vi "MPC_Sim_2.vi"() -> ()   [LabVIEW 2018]
uses:
  <vilib>/Simulation/Scripting/Companion Diagram/SimConfigNode/SimParams.ctl
  <vilib>/Simulation/Scripting/Companion Diagram/SimConfigNode/_simSolvers.ctl
  <vilib>/Simulation/Implementation/Shared/SIMSCR Execution Mode.ctl
  <vilib>/Simulation/Param Hierarchy/Typedefs/SIMPH Param Control Actions.ctl
  <vilib>/Simulation/Scripting/Editor Utilities/SIM subVI tag data.ctl
  <vilib>/Simulation/Scripting/Editor Utilities/SIM subVI execution type.ctl
  <vilib>/Simulation/Implementation/Shared/NILVSim_ParamChanged.vi
  <vilib>/Simulation/Implementation/Shared/NILVSIM_BeginStep.vi
  <vilib>/Simulation/Utility/Implementation/SIM Halt.vi
  <vilib>/Simulation/SignalArithmetic/Implementation/NILVSim Gain.llb/SIM Gain (vector).vi
  <vilib>/Simulation/Utility/Implementation/NILVSim Memory.llb/NILVSim Memory (core).vi
  <vilib>/Simulation/DiscreteLinear/Implementation/NILVSim Discrete State Space Buffered.llb/SIM Discrete State Space Distributor (SISO CD).vi
  <vilib>/Simulation/SignalArithmetic/Implementation/NILVSim Gain.llb/SIM Gain (scalar).vi
  <vilib>/Simulation/SignalDisplay/Implementation/NILVSim Time Waveform.llb/SIM Time Waveform (scalar).vi
  <vilib>/Simulation/Implementation/Shared/SIM Fire Discrete SubVI.vi
  <vilib>/Simulation/SignalDisplay/Implementation/NILVSim Time Waveform.llb/SIM Time Waveform (vector).vi
  <vilib>/Simulation/DiscreteLinear/Implementation/NILVSim Discrete State Space Buffered.llb/SIM Discrete State Space Collector (SISO CD).vi
  <vilib>/Simulation/Implementation/Shared/NILVSim_Manager.vi
  <vilib>/Utility/error.llb/Clear Errors.vi
  <vilib>/Simulation/Implementation/Shared/NILVSim_FinalizeModel.vi
  <vilib>/Simulation/Implementation/Shared/SIM Fire Discrete SubVI (Core).vi
  <vilib>/imath/engines/lvmath2/RunTimeEngine/IndexRead/NIMS M(S,S).vi
  <instcachedir>/0/NIMS M(S,S)_AC51E74150A542F7991B9634C66F3096.lvgen/NIMS M(S,S)_AC51E74150A542F7991B9634C66F3096_000.vi
  <vilib>/imath/engines/lvmath2/RunTimeEngine/IndexRead/NIMS V(S).vi
  <instcachedir>/0/NIMS V(S)_0488751826AF41519A22953C041130DC.lvgen/NIMS V(S)_0488751826AF41519A22953C041130DC_000.vi
  <vilib>/imath/engines/lvmath2/RunTimeEngine/IndexReplace/NIMS M(S,S)=S.vi
  <instcachedir>/0/NIMS M(S,S)=S_5DAF17B45D8A4C8588C7CF468644990A.lvgen/NIMS M(S,S)=S_5DAF17B45D8A4C8588C7CF468644990A_000.vi
  <vilib>/imath/engines/lvmath2/RunTimeEngine/ErrorHandling/NIMS_Create Error From Enums.vi
  <vilib>/imath/engines/lvmath/Plug In/Control Design/BuiltInFunctions/ss/NIMS_CD_ss(A,B,C,D).vi
  <vilib>/imath/engines/lvmath2/RunTimeEngine/NodeEndStatement/NIMS_NodeEndStatement_Output.vi
  <instcachedir>/0/NIMS_NodeEndStatement_Output_53EC0D466D134D7ABD903AC30B43404B.lvgen/NIMS_NodeEndStatement_Output_53EC0D466D134D7ABD903AC30B43404B_001.vi
  <instcachedir>/0/NIMS_NodeEndStatement_Output_53EC0D466D134D7ABD903AC30B43404B.lvgen/NIMS_NodeEndStatement_Output_53EC0D466D134D7ABD903AC30B43404B_011.vi
  <vilib>/imath/engines/lvmath2/RunTimeEngine/ErrorHandling/NIMS_Finalize Error.vi
  <vilib>/addons/Control Design/_Model Conversions/Continuous and Discrete.llb/Continuous and Discrete SubVI/cd_Convert Continuous to Discrete (SS).vi
  <vilib>/addons/Control Design/_MPC/Build Controller/CD Create MPC Controller (Barrier).vi
  <vilib>/imath/engines/lvmath2/RunTimeEngine/Managers/WorkSpace/UID Generator.vi
  <vilib>/imath/engines/lvmath2/RunTimeEngine/RangeToken/NIMS_Range.vi
  <instcachedir>/0/NIMS_Range_846134F467D14A349F7C6CCEF459CDB2.lvgen/NIMS_Range_846134F467D14A349F7C6CCEF459CDB2_000.vi
  <vilib>/imath/engines/lvmath2/RunTimeEngine/RunTimeType/NIMS_RunTimeType_From StrictType (excl LVString).vi
  <instcachedir>/0/NIMS_RunTimeType_From StrictType (excl LVString)_E7E34A65C99947108168652BAD14964D.lvgen/NIMS_RunTimeType_From StrictType (excl LVString)_E7E34A65C99947108168652BAD14964D_000.vi
  <vilib>/imathl/engines/lvmath/Functions/Error Handling/Create Error.vi
  <vilib>/imath/engines/lvmath2/RunTimeEngine/LocalVariableDefStatement/MC_LocalVariableDefStatement_Display.vi
  <vilib>/imath/engines/lvmath2/RunTimeEngine/BuiltInFunctions/square/NIMS_square.vi
  <instcachedir>/0/NIMS_square_8BE126634BDB49EE87F69273AACFE816.lvgen/NIMS_square_8BE126634BDB49EE87F69273AACFE816_001.vi
  <vilib>/imath/engines/lvmath2/RunTimeEngine/Managers/SymbolTable/Clear UID.vi
  <instcachedir>/0/NIMS_NodeEndStatement_Output_53EC0D466D134D7ABD903AC30B43404B.lvgen/NIMS_NodeEndStatement_Output_53EC0D466D134D7ABD903AC30B43404B_005.vi
  <vilib>/Simulation/Implementation/Shared/SIM Unbundle Sim Info.vi
  <vilib>/Simulation/Implementation/Shared/NILVSim_Initialize.vi
  <vilib>/Simulation/Utility/Implementation/NILVSim Get Time and IsAcceptedStep.vi
  <vilib>/addons/Control Design/_MPC/Reference Profile/CD Step Forward MPC Window.vi
  <vilib>/addons/Control Design/_MPC/Implement Controller/CD Implement MPC Controller.vi
  <vilib>/addons/Control Design/_MPC/Implement Controller/CD Implement MPC Controller (MIMO).vi
  <vilib>/Simulation/Implementation/Shared/SIMSH Read Queue.vi
  <vilib>/Simulation/Implementation/Shared/NILVSim_GetModelError.vi
  <vilib>/Simulation/Implementation/Shared/SIM Bundle Sim Info.vi
  <vilib>/Simulation/Scripting/Companion Diagram/SimConfigNode/SimDog.xnode
  <vilib>/addons/Control Design/_Model Construction/Model Typedefs.llb/CD State Space Model (MIMO).ctl
  <vilib>/addons/Control Design/_Model Construction/Model Typedefs.llb/CD General Elements.ctl
  <vilib>/Simulation/Implementation/XNodeFramework/SimXNode/SimX.xnode
  <vilib>/addons/Control Design/_Model Construction/NI_LinSys_Model Typedefs.lvlib
  <vilib>/addons/Control Design/_MPC/NI_CD_MPC.lvlib
  <vilib>/addons/Control Design/_Model Conversions/NI_CD_Continuous and Discrete.lvlib
  <vilib>/Simulation/DiscreteLinear/Implementation/NILVSim Discrete State Space Buffered.llb/SIM Discrete State Space Buffered (SISO CD).vi
  <vilib>/Simulation/Implementation/Shared/NI_SIM_Implementation.lvlib
  <vilib>/imath/engines/lvmath2/RunTimeEngine/Managers/SymbolTable/NIMS_WorkSpace.lvlib
panel:
  in  "Sampling Time":dbl=0.05 format="%#_13g"
  out "Loop Count":dbl=330.0
  out "Pendulum Min Angle":dbl
  out "Pendulum Max Angle":dbl
  out "Average distance from reference \nper sample (deg)":dbl
  out "t set":dbl[](array[numeric]) format="%#_13g"
  out "window":dbl[](array[numeric]) format="%#_13g"
  out "Pendulum Angle":waveform(dbl)(graph)
  out "Input and Tracking":waveform(dbl)[](graph)
  in  "Constraints (barrier)":T1
  out "Servo Voltage":waveform(dbl)(graph)
  in  "MPC Cost Weights":T2
  in  "MPC Controller Parameters":T3
  in  "Stop Button":bool
  in  "Frequency (Hz)":dbl=0.12500000000000003 min=0.005 max=1.0 step=0.005
  in  "Amplitude (deg)":dbl min=0.0 max=90.0 step=5.0
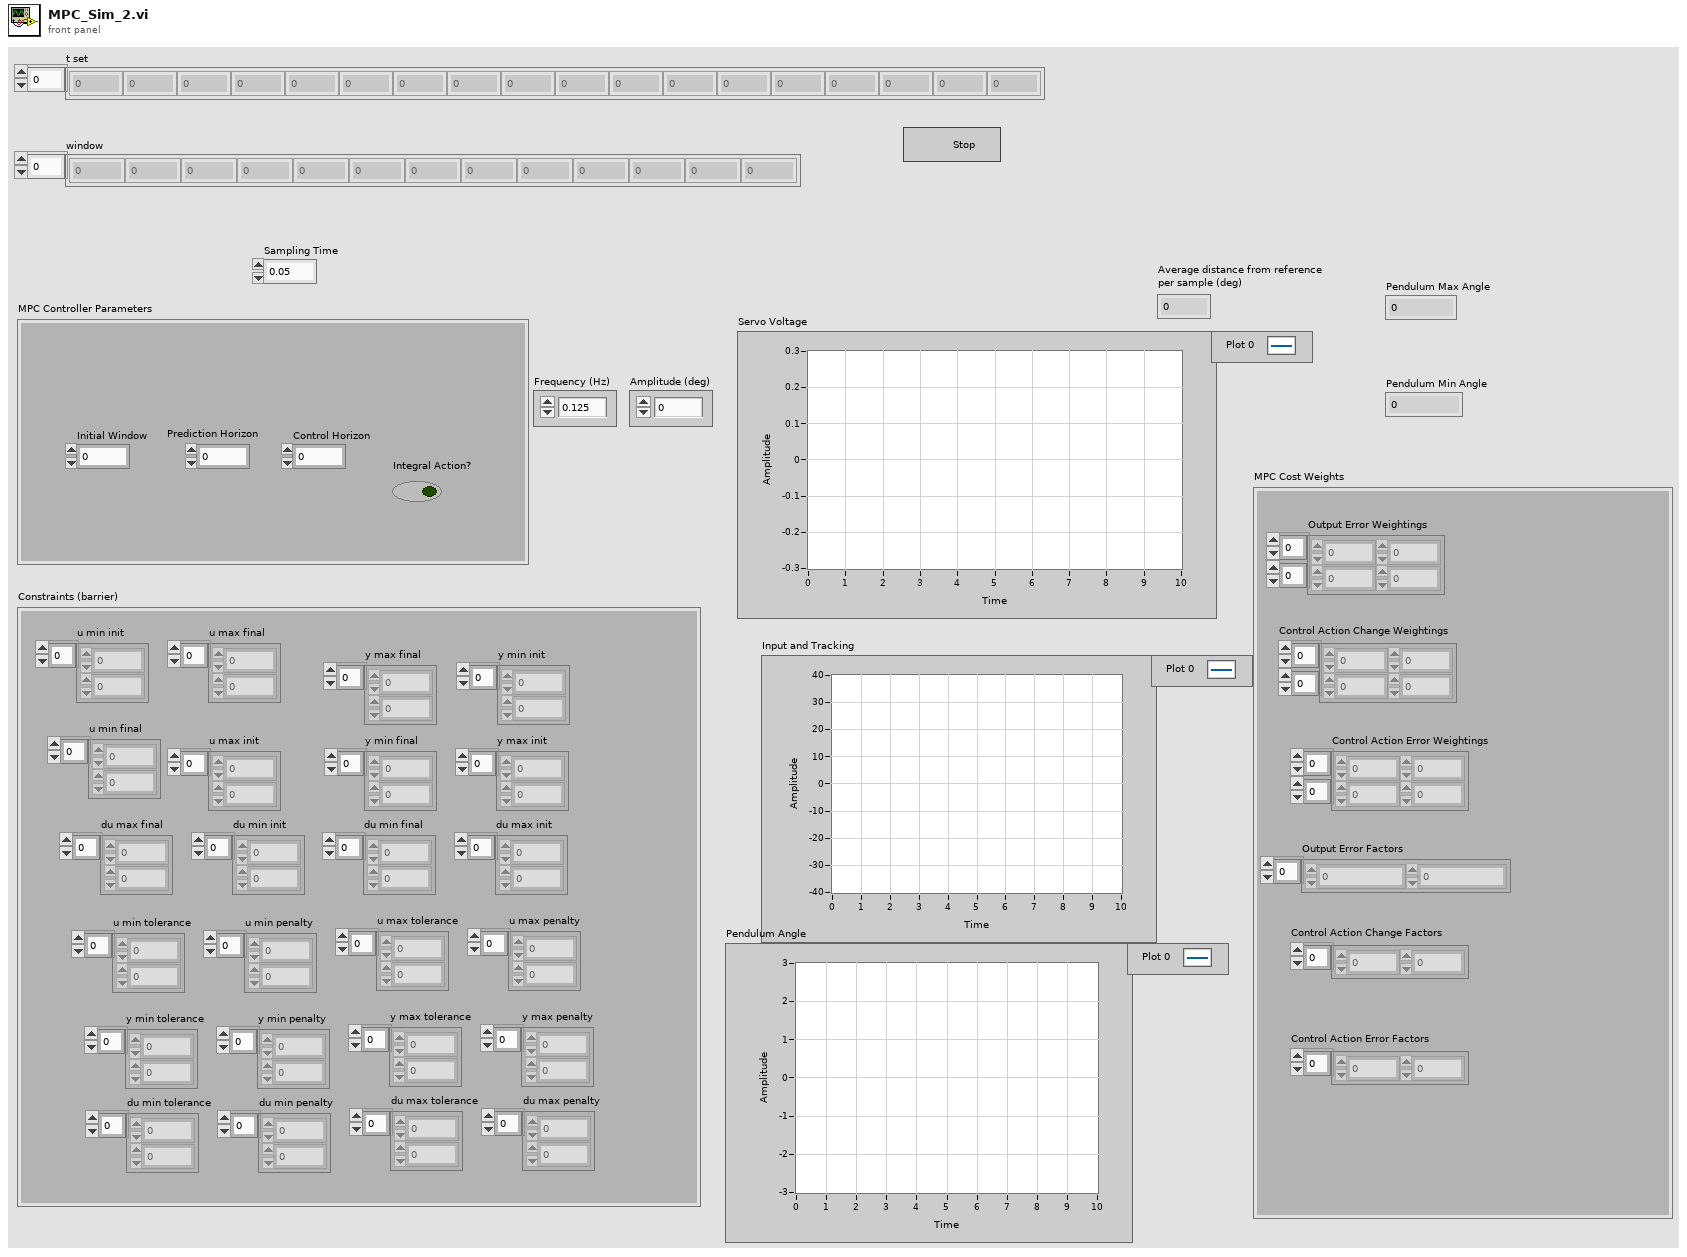
[diagram p1: front panel]
types:
  T1 = cluster{"u min init":dbl[], "u max final":dbl[], "u min final":dbl[], "u max init":dbl[], "y max final":dbl[], "y min init":dbl[], "y min final":dbl[], "y max init":dbl[], "du max final":dbl[], "du min init":dbl[], "du min final":dbl[], "du max init":dbl[], "u min tolerance":dbl[], "u min penalty":dbl[], "u max tolerance":dbl[], "u max penalty":dbl[], "y min tolerance":dbl[], "y min penalty":dbl[], "y max tolerance":dbl[], "y max penalty":dbl[], "du min tolerance":dbl[], "du min penalty":dbl[], "du max tolerance":dbl[], "du max penalty":dbl[]}
  T2 = cluster{"Output Error Weightings":dbl[][], "Control Action Change Weightings":dbl[][], "Control Action Error Weightings":dbl[][], "Output Error Factors":dbl[], "Control Action Change Factors":dbl[], "Control Action Error Factors":dbl[]}
  T3 = cluster{"Initial Window":i32, "Prediction Horizon":i32, "Control Horizon":i32, "Integral Action?":bool}
  T4 = typedef "NI_LinSys_Model Typedefs.lvlib/CD State Space Model (MIMO).ctl" = cluster{"properties":T5, "A":dbl[][], "B":dbl[][], "C":dbl[][], "D":dbl[][], "StateNames":string[], "Transport Delay":dbl[][]}
  T5 = typedef "NI_LinSys_Model Typedefs.lvlib/CD General Elements.ctl" = cluster{"Model name":string, "Input names":string[], "Output names":string[], "Input Delays":dbl[], "Output Delays":dbl[], "Sampling Time":dbl, "Notes":string}
  T6 = typedef "NI_CD_MPC.lvlib/CD MPC Model.ctl" = cluster{"H ":dbl[][], "G":dbl[][], "#Inputs":i32, "#Outputs":i32, "#States":i32, "#Disturbances":i32, "Integral Action?":bool, "Initial Data":T7, "Control Horizon":i32, "Prediction Horizon":i32, "Stopping Criteria":T8, "Inequality Constraints":T9, "Constraints":u16, "Initial Window":i32, "Internal Estimator?":bool, "L":dbl[][], "Plant Model (SS)":T4, "parameter bounds":cluster{"Xmin":dbl[], "Xmax":dbl[]}, "Sample Time":dbl, "Augmented SS Model":T4, "D":dbl[][], "K":dbl[][], "LN_y":dbl[][], "Inequality Constraints Barrier":T10, "H ^-1":dbl[][]}
  T7 = typedef "NI_CD_MPC.lvlib/CD MPC Data.ctl" = cluster{"Control Action (u)":dbl[], "Output (y)":dbl[], "Disturbance (d)":dbl[], "State (x)":dbl[], "Control Action Change (Du)":dbl[]}
  T8 = typedef "NI_Gmath.lvlib/stopping criteria.ctl" = cluster{"function tolerance":dbl, "parameter tolerance":dbl, "max iterations":i32, "max function calls":i32, "gradient tolerance":dbl, "max time (sec)":dbl}
  T9 = typedef "NI_CD_MPC.lvlib/CD Inequality Constraints and Parameter Bounds.ctl" = cluster{"Y max":dbl[], "Y min":dbl[], "U max":dbl[], "U min":dbl[], "tolerance":dbl}
  T10 = typedef "NI_CD_MPC.lvlib/CD Inequality Constraints and Parameter Bounds Barrier.ctl" = cluster{"Y max":dbl[], "Y min":dbl[], "U max":dbl[], "U min":dbl[], "dU max":dbl[], "dU min":dbl[], "pen min":dbl[], "tol min":dbl[], "pen max":dbl[], "tol max":dbl[]}
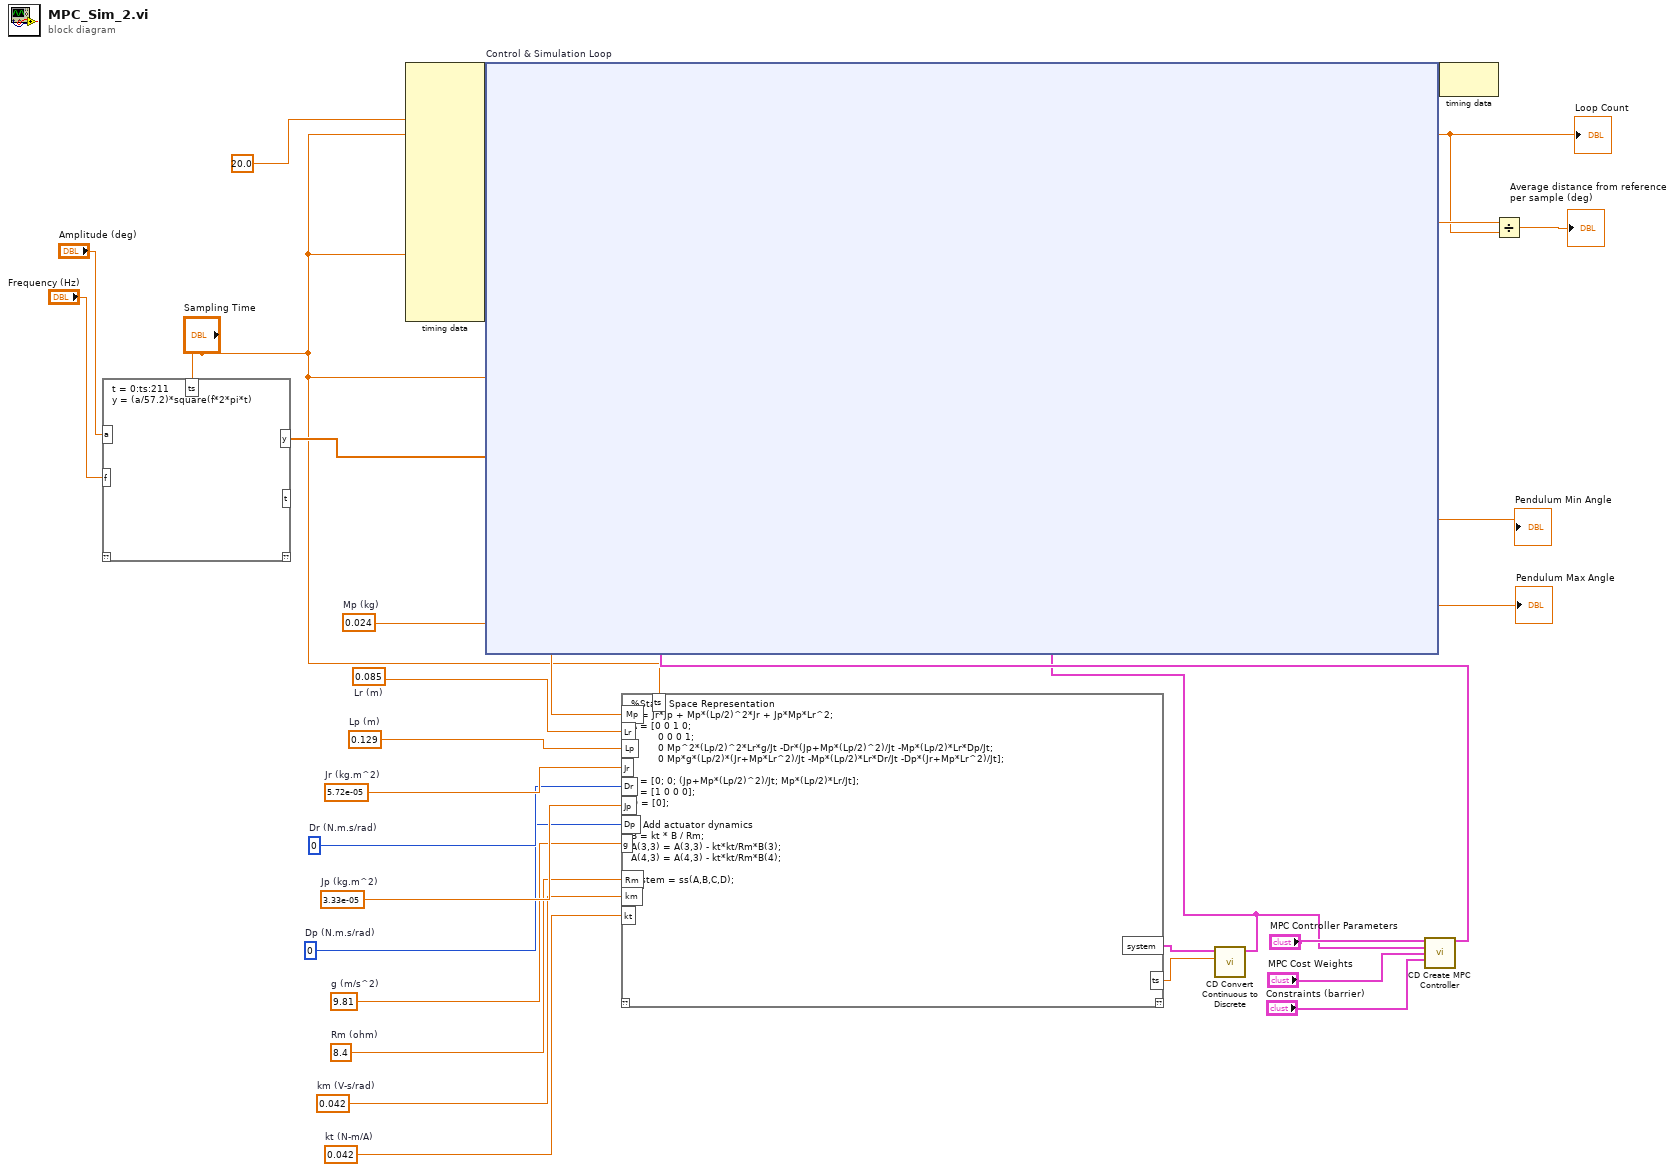
[diagram p0: block diagram]
diagram:
  w18 = 0.042  # kt (N-m/A)
  w19 = 0.042  # km (V-s/rad)
  w20 = 8.4  # Rm (ohm)
  w21 = 9.81  # g (m/s^2)
  w22 = 0  # Dp (N.m.s/rad)
  w23 = 3.33e-05  # Jp (kg.m^2)
  w24 = 0  # Dr (N.m.s/rad)
  w26 = 0.129  # Lp (m)
  w25 = 5.72e-05  # Jr (kg.m^2)
  w27 = 0.085  # Lr (m)
  w28 = 0.024  # Mp (kg)
  n1 = mathscript code="t = 0:ts:211\ny = (a/57.2)*square(f*2*pi*t)"("a"="Amplitude (deg)", "f"="Frequency (Hz)", "ts"="Sampling Time") -> ("y"=w11:dbl[])  [unwired: 1 in, 2 out]
  n2 = node-c288(20.0, "Sampling Time", "Sampling Time") -> (w30:variant)  [unwired: 13 in]
  n3 = mathscript code="%State Space Representation\nJt = Jr*Jp + Mp*(Lp/2)^2*Jr + Jp*Mp*Lr^2;\nA = [0 0 1 0;\n         0 0 0 1;\n         0 Mp^2*(Lp/2)^2*Lr*g/Jt -Dr*(Jp+Mp*(Lp/2)^2)/Jt -Mp*(Lp/2)*Lr*Dp/Jt;\n         0 Mp*g*(Lp/2)*(Jr+Mp*Lr^2)/Jt -Mp*(Lp/2)*Lr*Dr/Jt -Dp*(Jr+Mp*Lr^2)/Jt];\n\nB = [0; 0; (Jp+Mp*(Lp/2)^2)/Jt; Mp*(Lp/2)*Lr/Jt];\nC = [1 0 0 0];\nD = [0];\n\n% Add actuator dynamics\nB = kt * B / Rm;\nA(3,3) = A(3,3) - kt*kt/Rm*B(3);\nA(4,3) = A(4,3) - kt*kt/Rm*B(4);\n\nsystem = ss(A,B,C,D);"("Mp"=w28, "Lr"=w27, "Lp"=w26, "Jr"=w25, "Dr"=w24, "Jp"=w23, "Dp"=w22, "g"=w21, "Rm"=w20, "km"=w19, "kt"=w18, "ts"="Sampling Time") -> ("system"=w13:T4, "ts"=w12:dbl)  [unwired: 1 in, 1 out]
  n4 = call-poly <vilib>:"CD Convert Continuous to Discrete.vi"("Sampling Time (s)"=w12, "Continuous State-Space Model"=w13) -> ("Discrete State-Space Model"=w9:T4)  [unwired: 7 in, 2 out]
  n5 = call-poly <vilib>:"CD Create MPC Controller.vi"("MPC Controller Parameters"="MPC Controller Parameters", "State-Space Model"=w9, "MPC Cost Weights"="MPC Cost Weights", "MPC Constraints (Barrier)"="Constraints (barrier)") -> ("MPC Controller"=w14:T6)  [unwired: 10 in, 1 out]
  n6 = node-c254 "Control & Simulation Loop"(w30, w14, "Sampling Time", w11, w9) -> (w29:variant, w5:dbl, w4:dbl, →"Pendulum Min Angle":dbl, →"Pendulum Max Angle":dbl)
  "Loop Count" <- w4
  n7 = node-c288(w29) -> ()  [unwired: 1 out]
  n8 = Divide(x=w5, y=w4) -> (x/y=→"Average distance from reference \nper sample (deg)":dbl)
